vi "_test_validate_json_format.vi"() -> ()   [LabVIEW 2019, in "lv-apt-json-file-test.lvlib"]
uses:
  lv-apt-json-file-test.lvlib
  <vilib>/Utility/error.llb/Clear Errors.vi
  src/API/Json/Remove Comments.vi
  <userlib>/NEVSTOP-Programming-Palette/Configuration/Ini/TextToLines.vi
  <userlib>/_OpenG.lib/array/array.llb/Filter 1D Array__ogtk.vi
  <userlib>/_OpenG.lib/array/array.llb/Filter 1D Array (U8)__ogtk.vi
  <userlib>/NEVSTOP-Programming-Palette/Configuration/Ini/LinesToText.vi
  <vilib>/addons/_JKI.lib/Serialization/JSON/Library/Unflatten From JSON String.vi
  <vilib>/Utility/error.llb/Error Cluster From Error Code.vi
panel:
  out "error out":errorcluster
  out "String (dup)":string
  out "Json without comments":string
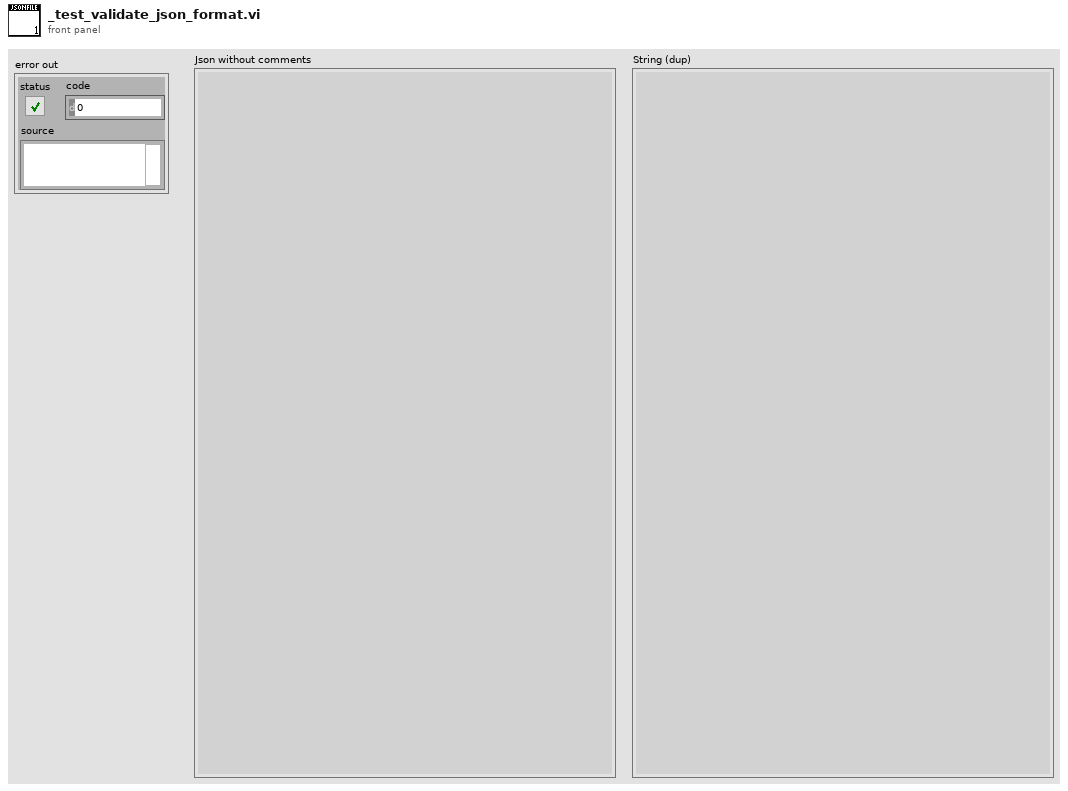
[diagram p1: front panel]
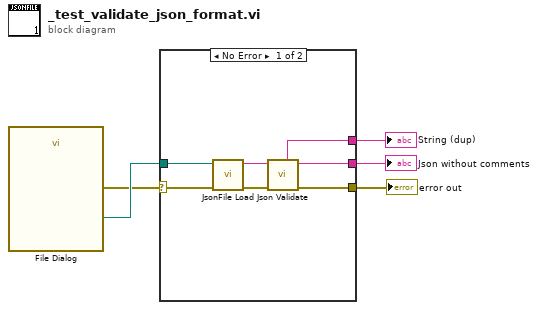
[diagram p0: block diagram]
diagram:
  n1 = call "File Dialog"() -> ("selected path"=w5:path, "error out"=w4:errorcluster)  [unwired: 12 in, 2 out]
  n2 = case shown="No Error" w4 {
    selector: w4 -> [w9 w13]
    tunnel: w5 -> [w10 _]
    tunnel: [w8 _] -> w2
    tunnel: [w7 _] -> w3
    tunnel: [w6 w13] -> w1
    frame No Error {
      n3 = call "JsonFile Load.vi"("error in (no error)"=w9, "Path"=w10) -> ("error out"=w11:errorcluster, "Json"=w12:string)  [unwired: 8 in]
      n4 = call "Json Validate.vi"("error in (no error)"=w11, "String"=w12) -> ("error out"=w6:errorcluster, "Json without comments"=w7:string, "String (dup)"=w8:string)  [unwired: 6 in, 1 out]
    }
    frame Error {
    }
  }
  "Json without comments" <- w3
  "String (dup)" <- w2
  "error out" <- w1
